vi "encode embedded message.vi"(10 "embedded message":u8[](array[numeric]), 11 "byte array in":u8[](array[numeric]) format="%.0b") -> (3 "byte array out":u8[](array[numeric]))   [LabVIEW 2013, in "protocol buffers encoder.lvlib"]
uses:
  protocol buffers encoder.lvlib
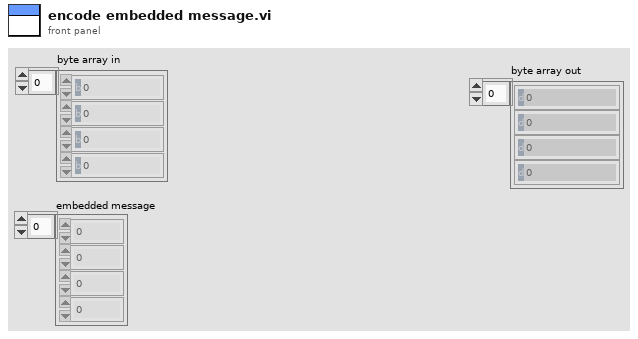
[diagram p1: front panel]
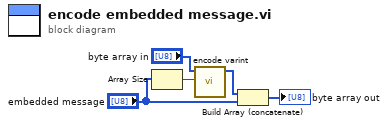
[diagram p0: block diagram]
diagram:
  n1 = Array Size(array="embedded message") -> (size(s)=w5:i32)
  n2 = call "encode varint.vi"("value"=w5, "byte array in"="byte array in") -> ("byte array out"=w3:u8[])  [unwired: 9 in]
  n3 = Build Array (concatenate)(w3, "embedded message") -> (→"byte array out":u8[])
